vi "WPI_PWMGetRangeScaleFactors.vi"(11 "DeadBand":T1) -> (1 "positiveScaleFactor":i32, 2 "negativeScaleFactor":i32, 3 "fullRangeScaleFactor":i32)   [LabVIEW 2017]
doc: "This software is licensed. Open the labview\\readme\\WPI Robotics Library Open Source License.txt file for more information."
uses:
  <vilib>/Rock Robotics/WPI/PWM/WPI_PWMDeadband.ctl
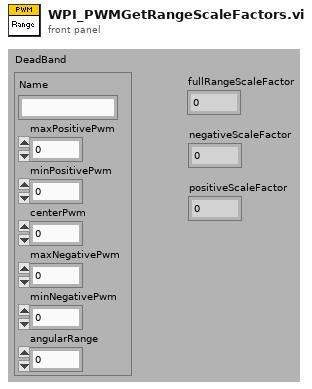
[diagram p1: front panel]
types:
  T1 = typedef "WPI_PWMDeadband.ctl" = cluster{"Name":string, "maxPositivePwm":i32, "minPositivePwm":i32, "centerPwm":i32, "maxNegativePwm":i32, "minNegativePwm":i32, "angularRange":u16}
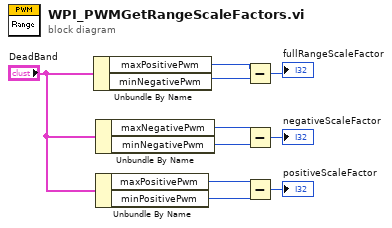
[diagram p0: block diagram]
diagram:
  n1 = Unbundle By Name("DeadBand") -> ("maxPositivePwm"=w10:i32, "minNegativePwm"=w9:i32)
  n2 = Unbundle By Name("DeadBand") -> ("maxNegativePwm"=w5:i32, "minNegativePwm"=w6:i32)
  n3 = Unbundle By Name("DeadBand") -> ("maxPositivePwm"=w2:i32, "minPositivePwm"=w3:i32)
  n4 = Subtract(x=w10, y=w9) -> (x-y=→"fullRangeScaleFactor":i32)
  n5 = Subtract(x=w5, y=w6) -> (x-y=→"negativeScaleFactor":i32)
  n6 = Subtract(x=w2, y=w3) -> (x-y=→"positiveScaleFactor":i32)
